vi "FileFunctions.ReadFirstAndLastLine.vi"(8 "error in":errorcluster, 10 "Aprox. StringLength":i32, 11 "selected path":path) -> (0 "error out":errorcluster, 1 "LastRow":string[](array[string]), 2 "First Row":string[](array[string]), 3 "Header":string[](array[string]), 4 "SignalCount":i32, 5 "TwoSubsequentRows":string[][](array[string]), 6 "FileSize(Bytes)":i64, 7 "Delimiter":string)   [LabVIEW 2016]
uses:
  <vilib>/dlg_ctls.llb/Space Constant.vi
  <vilib>/Utility/error.llb/Search and Replace Pattern.vi
  <vilib>/Utility/error.llb/Trim Whitespace.vi
  <vilib>/Utility/file.llb/Read Delimited Spreadsheet (string).vi
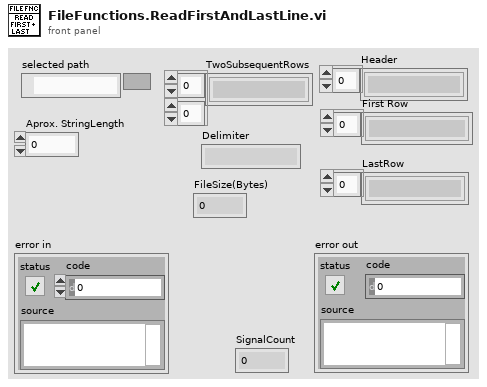
[diagram p1: front panel]
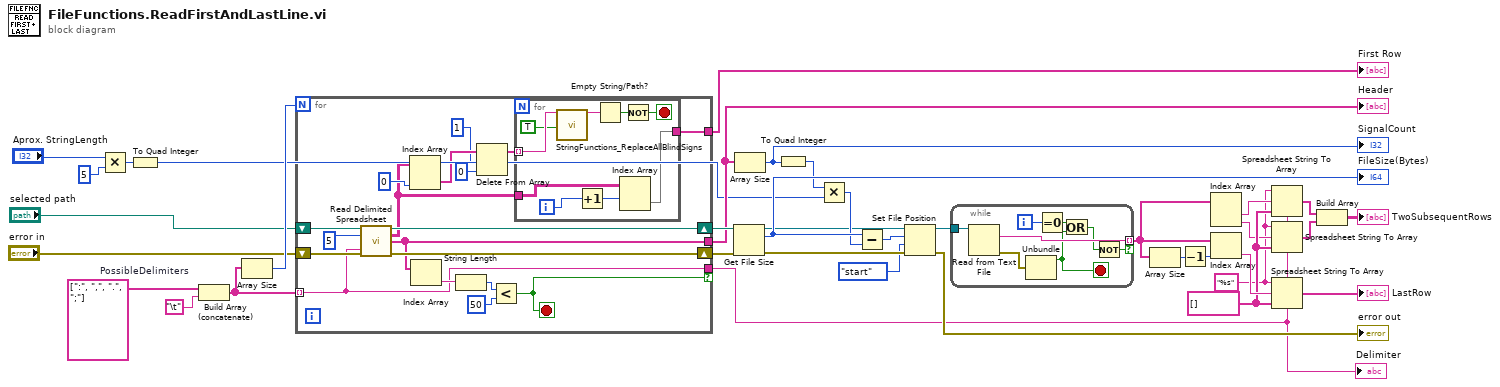
[diagram p0: block diagram]
diagram:
  w5 = "%s" ("format string")
  w8 = string[] [] ("type (empty)")
  w35 = string[] [":", ",", ".", ";"]  # PossibleDelimiters
  n1 = Multiply(x="Aprox. StringLength", y=5) -> (x*y=w21:i32)
  n2 = To Quad Integer(1:w21) -> (0:w12:i64)
  n3 = Build Array (concatenate)(w35, "\t") -> (w36:string[])
  n4 = Array Size(array=w36) -> (size(s)=w37:i32)
  n5 = for {
    N: w37 -> [_]
    shift-right: [w53] -> w17
    shift-left: "error in" -> [w55]
    tunnel: w36 -> [w49] mode=indexing
    tunnel: [w49] -> w4 if=w47
    shift-right: [w46] -> w23
    shift-left: "selected path" -> [w54]
    tunnel: [w45] -> w14
    tunnel: [w38] -> w11
    stop <- w47 stop-if-true
    n6 = call-poly <vilib>:"Read Delimited Spreadsheet.vi"("file path (dialog if empty)"=w54, "number of rows (all:-1)"=5, "error in (no error)"=w55, "delimiter (\\t)"=w49) -> ("new file path (Not A Path if cancelled)"=w46:path, "all rows"=w39:string[][], "first row"=w45:string[], "error out"=w53:errorcluster)  [unwired: 6 in, 2 out]
    n7 = Index Array(array=w39, index (col)=0 ("disabled index (col)")) -> (element=w43:string[])  [unwired: 1 in]
    n8 = Index Array(array=w45) -> (element=w50:string)  [unwired: 1 in]
    n9 = String Length(string=w50) -> (length=w52:i32)
    n10 = Delete From Array(array=w43, length=1, index=0) -> (array with subset deleted=w40:string[])  [unwired: 1 out]
    n11 = Less?(x=w52, y=50) -> (x < y?=w47:bool)
    n12 = for {
      tunnel: w40 -> [w58] mode=indexing
      tunnel: w39 -> [w62]
      tunnel: [w61] -> w38
      i -> [w59]
      stop <- w63 stop-if-true
      n13 = call "StringFunctions_ReplaceAllBlindSigns.vi"("String"=w58, "RemoveSpaceAswell"=TRUE) -> ("ModifiedString"=w56:string)  [unwired: 16 in, 1 out]
      n14 = Increment(x=w59) -> (x+1=w60:i32)
      n15 = Empty String/Path?(string/path=w56) -> (empty?=w64:bool)
      n16 = Index Array(array=w62, index (row)=w60) -> (element=w61:string[])  [unwired: 1 in]
      n17 = Not(x=w64) -> (.not. x?=w63:bool)
    }
  }
  "Header" <- w14
  "First Row" <- w11
  "Delimiter" <- w4
  n18 = Get File Size(file=w23, error in=w17) -> (refnum out=w22:refnum<file>, size (in bytes)=w33:i64, 0:w19:errorcluster)
  "FileSize(Bytes)" <- w33
  n19 = Array Size(array=w14) -> (size(s)=w32:i32)
  "SignalCount" <- w32
  n20 = To Quad Integer(1:w32) -> (0:w20:i64)
  n21 = Multiply(x=w20, y=w12) -> (x*y=w31:i64)
  n22 = Subtract(x=w33, y=w31) -> (x-y=w30:i64)
  n23 = Set File Position(offset (in bytes) (0)=w30, refnum=w22, from (0:start)=enum16{"start", "end", "current"}."start", error in=w19) -> (refnum out=w29:refnum<file>, error out=→"error out":errorcluster)
  n24 = while {
    tunnel: w29 -> [w72]
    tunnel: [w69] -> w9 mode=indexing if=w70
    i -> [w68]
    stop <- w66 stop-if-true
    n25 = Read from Text File(file (use dialog)=w72) -> (text=w69:string, error out=w71:errorcluster)  [unwired: 3 in, 2 out]
    n26 = Unbundle(w71) -> ("status"=w66:bool)  [unwired: 2 out]
    n27 = Equal To 0?(x=w68) -> (x = 0?=w67:bool)
    n28 = Or(x=w67, y=w66) -> (x .or. y?=w65:bool)
    n29 = Not(x=w65) -> (.not. x?=w70:bool)
  }
  n30 = Array Size(array=w9) -> (size(s)=w28:i32)
  n31 = Decrement(x=w28) -> (x-1=w10:i32)
  n32 = Index Array(array=w9) -> (element #1=w7:string, element #2=w6:string)  [unwired: 2 in]
  n33 = Index Array(array=w9, index=w10) -> (element=w16:string)
  n34 = Spreadsheet String To Array(delimiter (Tab)=w4, format string=w5, spreadsheet string=w7, array type (2D Dbl)=w8) -> (array=w2:string[])
  n35 = Spreadsheet String To Array(delimiter (Tab)=w4, format string=w5, spreadsheet string=w6, array type (2D Dbl)=w8) -> (array=w3:string[])
  n36 = Spreadsheet String To Array(delimiter (Tab)=w4, format string=w5, spreadsheet string=w16, array type (2D Dbl)=w8) -> (array=→"LastRow":string[])
  n37 = Build Array(w2, w3) -> (→"TwoSubsequentRows":string[][])
